vi "3_AdvancedDemo_MHT3.vi"() -> ()   [LabVIEW 2017]
uses:
  Types/MH_InputChannel.ctl
  Types/MH_UIThread_Cmds.ctl
  Types/MH_UIThread_Data.ctl
  _lib/PQ/MultiHarp/MH_InitInfo.ctl
  Types/MH_SetInpChanData.ctl
  Types/MH_SetInpChanCmds.ctl
  Types/MH_DataProcThread_QData.ctl
  Types/MH_DataProcThread_QCmds.ctl
  Types/MH_VisThread_QData.ctl
  Types/MH_VisThread_QCmds.ctl
  Types/MH_VisThread_Data.ctl
  _lib/PQ/MultiHarp/MH_RefSource.ctl
  _lib/PQ/MultiHarp/MH_MeasMode.ctl
  <vilib>/Utility/error.llb/DialogType.ctl
  <vilib>/Utility/error.llb/Error Cluster From Error Code.vi
  _lib/PQ/MultiHarp/MH_LibVersion_global.vi
  _lib/PQ/MultiHarp/mhlib_x86_x64_UIThread.llb/MH_DllPath_global.vi
  <vilib>/ErrorRing/Error Ring.xnode
panel:
  in  "Settings":bool=TRUE
  in  "Run continuously":bool caption="Conti."
  in  "Start":bool
  in  "Scale":bool
  out "CountRates":i32[](graph)
  in  "AllChannels":T1={"Enable"=TRUE, "Offset"=0, "Level"=-100, "Edge"=0, "DeadTime"=1000, "UseDeadTime"=FALSE, "SetEnableAllChan"=TRUE, "SetEdgeAllChan"=TRUE, "SetLevelAllChan"=TRUE, "SetOffsetAllChan"=TRUE, "SetUseDTAllChan"=TRUE, "SetDeadTAllChan"=TRUE} {"DeadTime" min=800 max=160000 step=1; "Edge" items=["falling", "rising"]; "Offset" min=-100000 max=100000 step=80; "Level" min=-1200 max=1200 step=1}
  in  "HistoAcqTime":dbl=1.0 caption="Hist.Int.Time  s" min=0.1 max=360000.0 step=0.1
  in  "AcqTime":i32=360000000 caption="T3Acqu.       ms" min=1 max=360000 step=1
  in  "Binning":i32(ring) caption="Resol.            ps" items=["80", "160", "320", "640", "1280", "2560", "5120", "10240", "20480", "40960", "81920", "163840", "327680", "655360", "1310720", "2621440", "5242880", "10485760", "20971520", "41943040", "83886080", "167772160", "335544320"]
  in  "HistoOffset":i32 caption="Offset            ns" min=0 max=100000000 step=1
  out "DeltaT":dbl=6.553665536655367 caption="T.Tr.Resol.   ms" format="%.2f"
  in  "BitShift":i32=15 min=0 max=32 step=1
  in  "OvlLevel":u32=4294967295 caption="Ovl.Level" min=1024 max=65536 step=1024
  in  "StopOvl.":bool=TRUE
  out "TTraceGraph":T2(graph)={49.38852226226715, "Resolution"=0.00655367864414373, "Histogram"=[]}
  out "HistoGraph":cluster{dbl, "Resol":dbl, "Histos":u32[][]}(graph)={0.0, "Resol"=0.08, "Histos"=[]}
  in  "SyncDeadTime":i32=1000 caption="Dead T.   ps" min=800 max=160000 step=1
  in  "UseDeadTime":bool caption="Use DT."
  in  "SyncEdge":i32(ring) caption="Edge" items=["falling", "rising"]
  in  "SyncDivider":i32(ring) caption="Divider" items=["1", "2", "4", "8", "16"]
  in  "SyncOffset":i32 caption="Offset      ps" min=-100000 max=100000 step=80
  in  "SyncLevel":i32=-100 caption="Level      mV" min=-1200 max=1200 step=1
  in  "Channels":T3[](array[typedef])=[{"Name"="Inp.Chan 1", "Enable"=TRUE, "Edge"=0, "Level"=-100, "Offset"=0, "UseDeadTime"=FALSE, "DeadTime"=1000}, {"Name"="Inp.Chan 2", "Enable"=TRUE, "Edge"=0, "Level"=-100, "Offset"=0, "UseDeadTime"=FALSE, "DeadTime"=1000}, {"Name"="Inp.Chan 3", "Enable"=TRUE, "Edge"=0, "Level"=-100, "Offset"=0, "UseDeadTime"=FALSE, "DeadTime"=1000}, {"Name"="Inp.Chan 4", "Enable"=TRUE, "Edge"=0, "Level"=-100, "Offset"=0, "UseDeadTime"=FALSE, "DeadTime"=1000}, {"Name"="Inp.Chan 5", "Enable"=TRUE, "Edge"=0, "Level"=-100, "Offset"=0, "UseDeadTime"=FALSE, "DeadTime"=1000}, {"Name"="Inp.Chan 6", "Enable"=TRUE, "Edge"=0, "Level"=-100, "Offset"=0, "UseDeadTime"=FALSE, "DeadTime"=1000}, {"Name"="Inp.Chan 7", "Enable"=TRUE, "Edge"=0, "Level"=-100, "Offset"=0, "UseDeadTime"=FALSE, "DeadTime"=1000}, {"Name"="Inp.Chan 8", "Enable"=TRUE, "Edge"=0, "Level"=-100, "Offset"=0, "UseDeadTime"=FALSE, "DeadTime"=1000}, {"Name"="Inp.Chan 9", "Enable"=TRUE, "Edge"=0, "Level"=-100, "Offset"=0, "UseDeadTime"=FALSE, "DeadTime"=1000}, {"Name"="Inp.Chan 10", "Enable"=TRUE, "Edge"=0, "Level"=-100, "Offset"=0, "UseDeadTime"=FALSE, "DeadTime"=1000}, {"Name"="Inp.Chan 11", "Enable"=TRUE, "Edge"=0, "Level"=-100, "Offset"=0, "UseDeadTime"=FALSE, "DeadTime"=1000}, {"Name"="Inp.Chan 12", "Enable"=TRUE, "Edge"=0, "Level"=-100, "Offset"=0, "UseDeadTime"=FALSE, "DeadTime"=1000}, {"Name"="Inp.Chan 13", "Enable"=TRUE, "Edge"=0, "Level"=-100, "Offset"=0, "UseDeadTime"=FALSE, "DeadTime"=1000}, {"Name"="Inp.Chan 14", "Enable"=TRUE, "Edge"=0, "Level"=-100, "Offset"=0, "UseDeadTime"=FALSE, "DeadTime"=1000}, {"Name"="Inp.Chan 15", "Enable"=TRUE, "Edge"=0, "Level"=-100, "Offset"=0, "UseDeadTime"=FALSE, "DeadTime"=1000}, {"Name"="Inp.Chan 16", "Enable"=TRUE, "Edge"=0, "Level"=-100, "Offset"=0, "UseDeadTime"=FALSE, "DeadTime"=1000}] {"DeadTime" min=800 max=160000 step=1; "Edge" items=["falling", "rising"]; "Offset" min=-100000 max=100000 step=80; "Level" min=-1200 max=1200 step=1}
  out "SyncRate":string="Sync Rate: 4999940 cps\n"
  out "OverRun":bool caption="Overrun:"
  out "Status":string="Elements in Q: 0"
  # "All Channels"
  # "Acquisition"
  # "Sync"
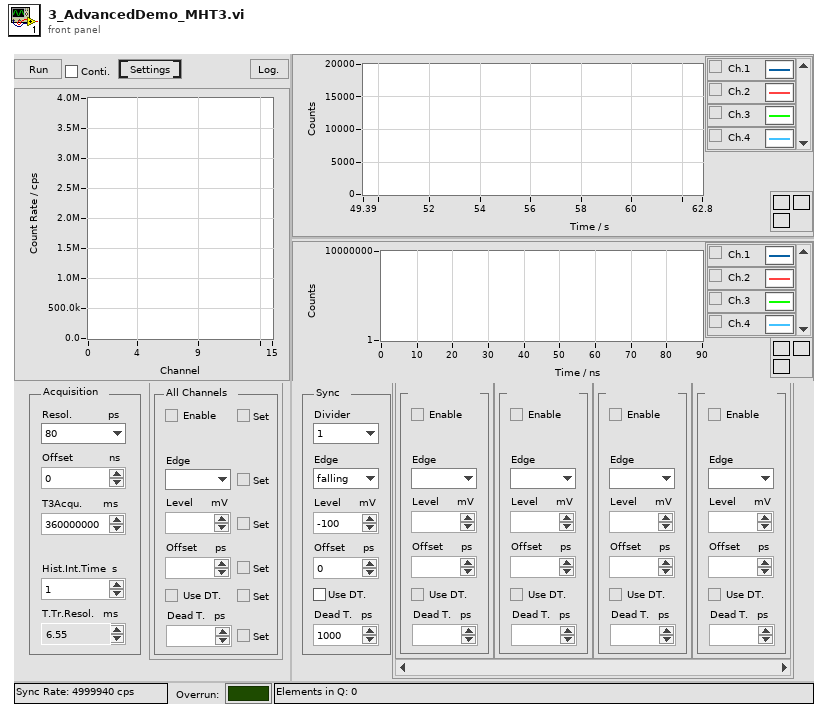
[diagram p1: front panel]
types:
  T1 = cluster{"Enable":bool, "Offset":i32, "Level":i32, "Edge":i32, "DeadTime":i32, "UseDeadTime":bool, "SetEnableAllChan":bool, "SetEdgeAllChan":bool, "SetLevelAllChan":bool, "SetOffsetAllChan":bool, "SetUseDTAllChan":bool, "SetDeadTAllChan":bool}
  T2 = cluster{dbl, "Resolution":dbl, "Histogram":u32[][]}
  T3 = typedef "MH_InputChannel.ctl" = cluster{"Name":string, "Enable":bool, "Edge":i32, "Level":i32, "Offset":i32, "UseDeadTime":bool, "DeadTime":i32}
  T4 = typedef "MH_DataProcThread_QCmds.ctl" = enum16{"Exit", "Proc", "Init", "SetShift", "SetNumChannels", "SetHistAcqTime"}
  T5 = typedef "MH_VisThread_Data.ctl" = cluster{"Resol":dbl, "DeltaT":dbl, "NumChannels":i32}
  T6 = typedef "MH_VisThread_QData.ctl" = cluster{"Histos":u32[][], "Cmd":T7, "TimeTrace":u32[][], "Bin":i32, "Total bin":u64, "Status":string, "Resol":dbl, "DeltaT":dbl, "nChannels":i32}
  T7 = typedef "MH_VisThread_QCmds.ctl" = enum16{"_none_", "Resol", "nChannels", "DeltaT", "Histo", "TTrace", "Status"}
  T8 = typedef "MH_DataProcThread_QData.ctl" = cluster{"Cmd":T4, "nActual":i32, "Buffer":u32[], "TickCount":u32, "Param":i32}
  T9 = typedef "MH_UIThread_Data.ctl" = cluster{"Init Info":T10, "DevIdx":i32, "SyncDivider":i32, "SyncOffset":i32, "SyncLevel":i32, "Channels":T3[], "CurrentChannels":i32[], "AcqTime":i32, "Binning":i32, "HistoOffset":i32, "HistoLen":i32, "StopOvl.":bool, "OvlLevel":u32, "SyncEdge":i32, "StartMeas":bool, "HistoLength":i32, "Resolution":dbl, "Run cont.":bool, "Status":string, "SyncRate":i32, "BitShift":i32, "HistoAcqTime":dbl, "SyncRateStart":i32, "UseDeadTime":bool, "SyncDeadTime":i32, "SetInpChan":T11[]}
  T10 = typedef "MH_InitInfo.ctl" = cluster{"Library Version":string, "Serial No.":string, "Model":string, "Partnum":string, "Version":string, "features":i32, "nchannels":i32, "Base Resolution":dbl, "Bin Steps":i32}
  T11 = typedef "MH_SetInpChanData.ctl" = cluster{"Channel":i32, "Cmds":T12[], "Changed":cluster{"Name":bool, "Enable":bool, "Edge":bool, "Level":bool, "Offset":bool, "UseDeadTime":bool, "DeadTime":bool}}
  T12 = typedef "MH_SetInpChanCmds.ctl" = enum16{"SetInpChanEnable", "SetInpChanOffset", "SetInpChanDeadTime", "SetInpChanTrg"}
  T13 = typedef "MH_UIThread_Cmds.ctl" = enum16{"Idle", "Init", "SetInpChan", "SetSyncDivider", "SetSyncTrg", "SetSyncOffset", "SetSyncDeadTime", "SetBinning", "SetHistoOffset", "SetHistoLen", "SetStopOvl", "SetBitShift", "SetHistoAcqTime", "GetRates", "GetAllRates", "StartMeas", "StopMeas", "AbortMeas", "GetResolution", "GetHistos", "GetAllHistos", "ReadFiFo", "WriteStatus", "Resize", "EnableControls", "DisableControls", "Error", "Exit"}
  T14 = enum8{"Enabled", "Disabled", "Disabled and Grayed Out"}
  T15 = cluster{"[0]":bool, "[1]":bool, "[2]":bool, "[3]":bool, "[4]":bool, "[5]":bool}
  T16 = typedef "MH_MeasMode.ctl" = i32
  T17 = typedef "MH_RefSource.ctl" = enum16{"INTERNAL", "EXTERNAL_10MHZ", "WR_MASTER_GENERIC", "WR_SLAVE_GENERIC", "WR_GRANDM_GENERIC", "EXTN_GPS_PPS", "EXTN_GPS_PPS_UART", "WR_MASTER_MHARP", "WR_SLAVE_MHARP", "WR_GRANDM_MHARP"}
  T18 = typedef "DialogType.ctl" = u16
  T19 = cluster{"T0":dbl, "dt":dbl, "TimeTrace_out":u32[][]}
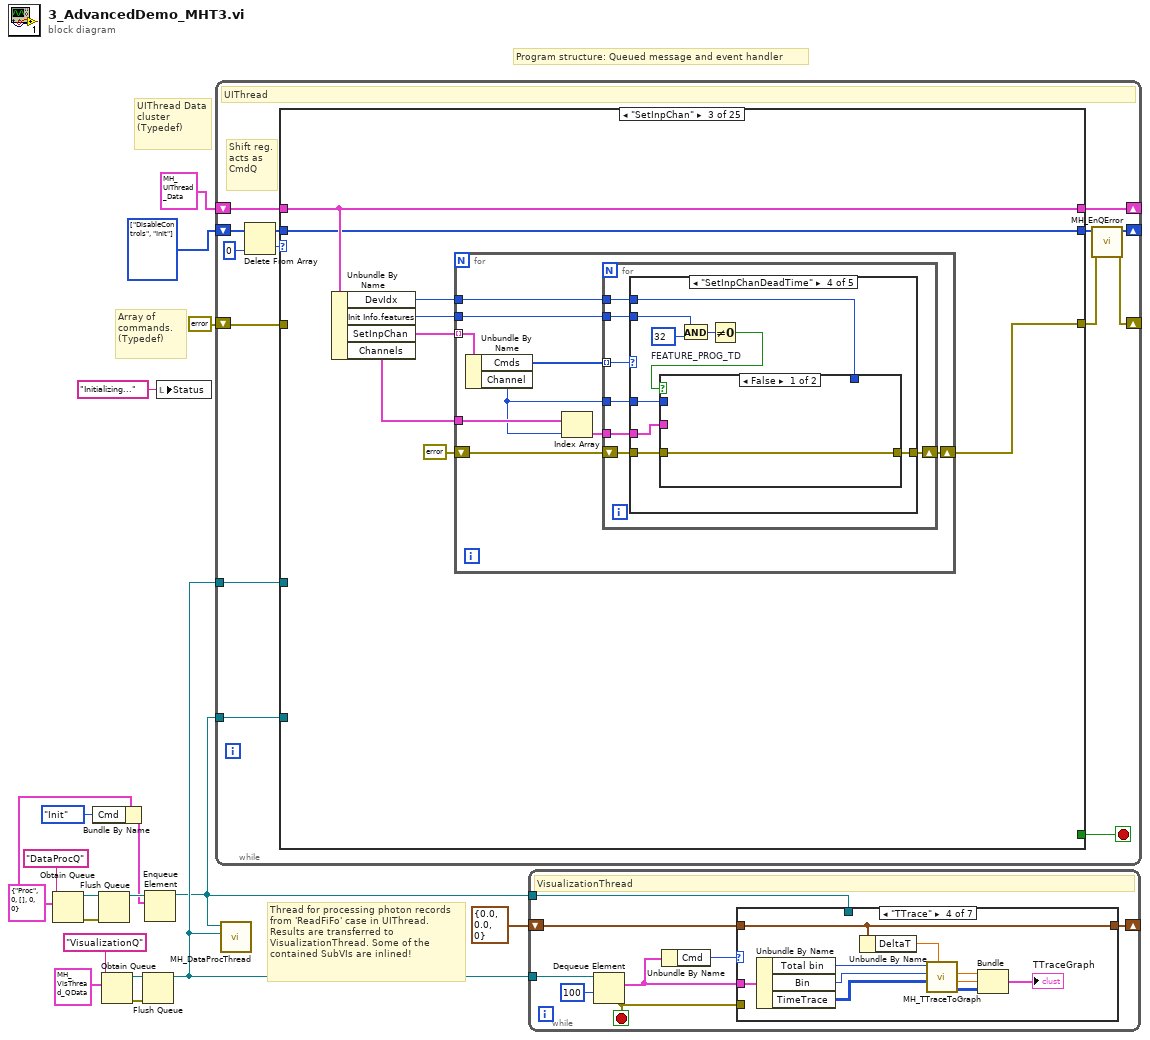
[diagram p0: block diagram]
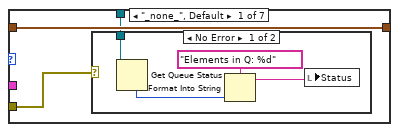
[diagram p2: hidden frame]
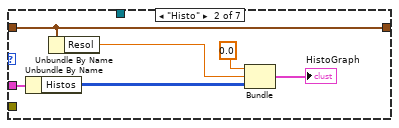
[diagram p4: hidden frame]
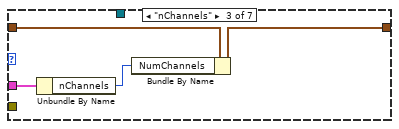
[diagram p5: hidden frame]
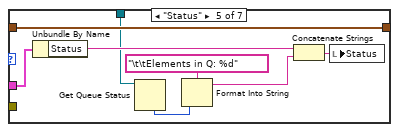
[diagram p6: hidden frame]
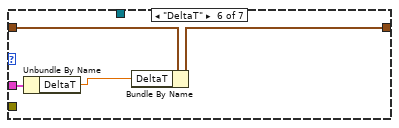
[diagram p7: hidden frame]
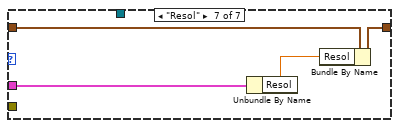
[diagram p8: hidden frame]
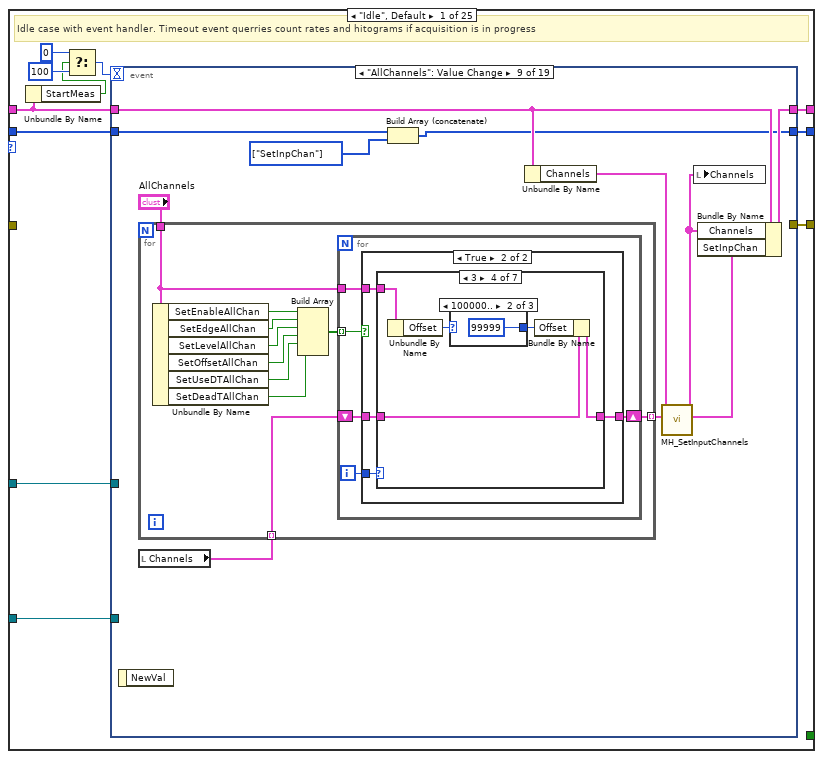
[diagram p9: hidden frame]
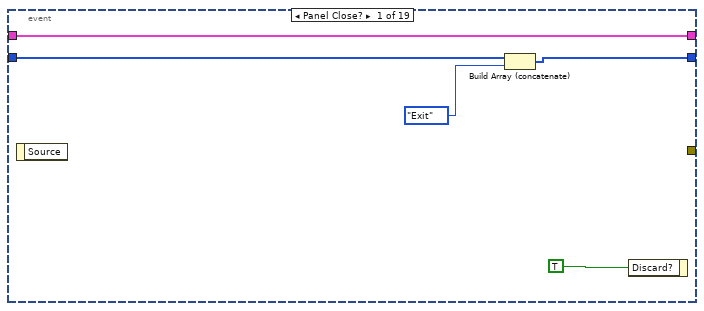
[diagram p10: hidden frame]
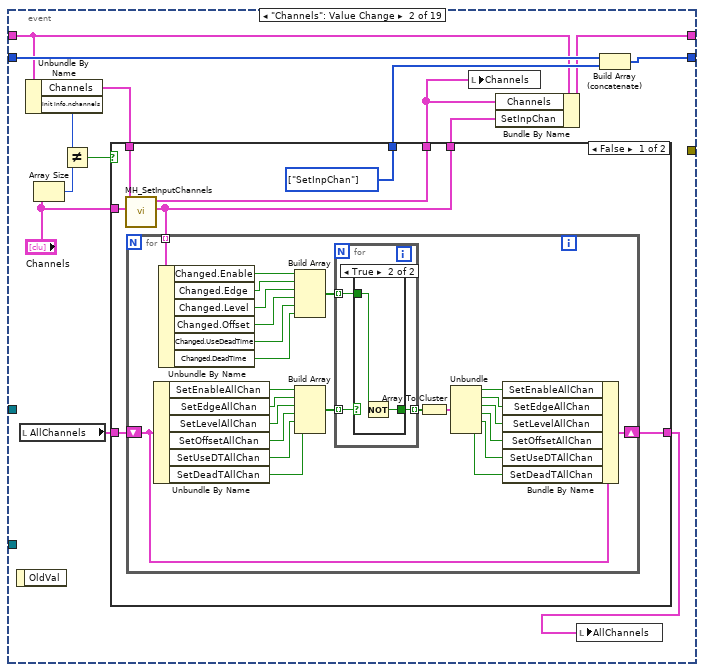
[diagram p11: hidden frame]
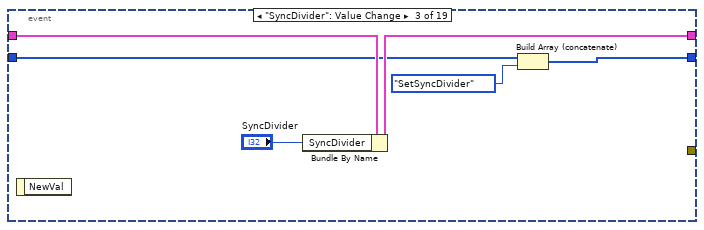
[diagram p14: hidden frame]
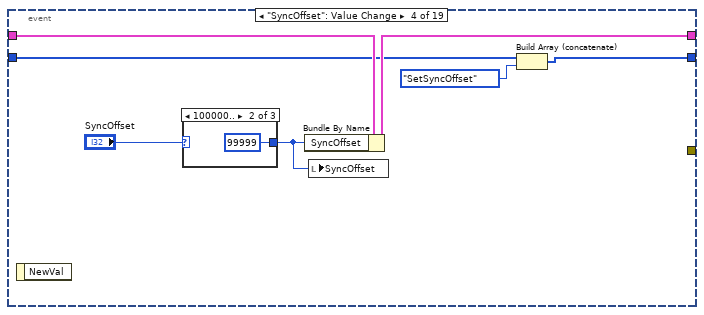
[diagram p15: hidden frame]
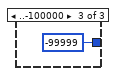
[diagram p17: hidden frame]
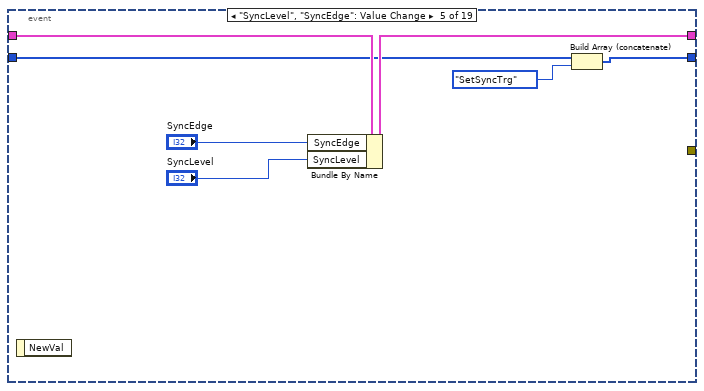
[diagram p18: hidden frame]
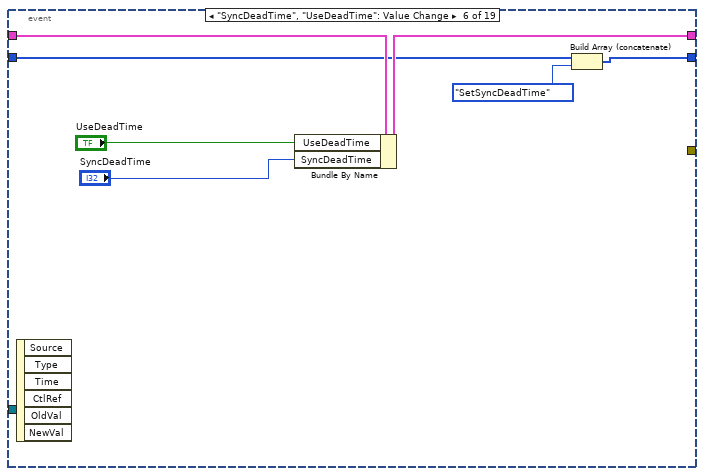
[diagram p19: hidden frame]
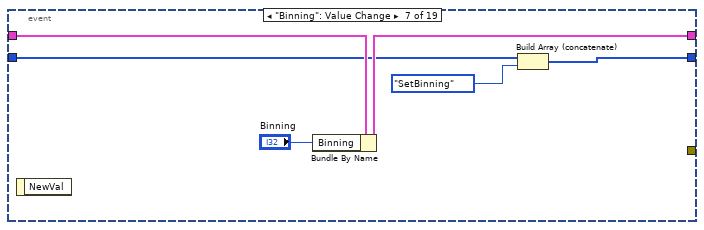
[diagram p20: hidden frame]
diagram:
  w4 = T8 {"Cmd"=enum."Proc", "nActual"=0, "Buffer"=[], "TickCount"=0, "Param"=0} ("MH_DataProcThread_QData")
  w17 = T13[] [enum."DisableControls", enum."Init"] items=["Idle", "Init", "SetInpChan", "SetSyncDivider", "SetSyncTrg", "SetSyncOffset", "SetSyncDeadTime", "SetBinning", "SetHistoOffset", "SetHistoLen", "SetStopOvl", "SetBitShift", "SetHistoAcqTime", "GetRates", "GetAllRates", "StartMeas", "StopMeas", "AbortMeas", "GetResolution", "GetHistos", "GetAllHistos", "ReadFiFo", "WriteStatus", "Resize", "EnableControls", "DisableControls", "Error", "Exit"]
  # "Thread for processing photon records from 'ReadFiFo' case in UIThread. Results are transferred to VisualizationThread. Some of the contained SubVIs are inlined!"
  # "Array of commands.\n(Typedef)"
  # "Program structure: Queued message and event handler"
  # "UIThread Data cluster\n(Typedef)"
  n1 = Obtain Queue(name (unnamed)="DataProcQ", element data type=w4) -> (queue out=w14:refnum<queue>, error out=w13:errorcluster)  [unwired: 3 in, 1 out]
  n2 = Bundle By Name(cluster=w4, "Cmd"=MH_DataProcThread_QCmds."Init") -> (w2:T8)
  n3 = Flush Queue(queue=w14, error in (no error)=w13) -> (queue out=w5:refnum<queue>)  [unwired: 2 out]
  n4 = Obtain Queue(name (unnamed)="VisualizationQ", element data type=T6 {"Histos"=[], "Cmd"=enum."_none_", "TimeTrace"=[], "Bin"=0, "Total bin"=0, "Status"="", "Resol"=0.0, "DeltaT"=0.0, "nChannels"=0} ("MH_GUIThread_QData")) -> (queue out=w12:refnum<queue>, error out=w11:errorcluster)  [unwired: 3 in, 1 out]
  n5 = Flush Queue(queue=w12, error in (no error)=w11) -> (queue out=w7:refnum<queue>)  [unwired: 2 out]
  n6 = Enqueue Element(queue=w5, element=w2) -> (queue out=w1:refnum<queue>)  [unwired: 2 in, 2 out]
  n7 = local write "Status"("Initializing..." ("Status")) -> ()
  n8 = while {
    shift-right: [w21] -> _
    shift-left: w17 -> [w28]
    shift-right: [w31] -> _
    shift-left: T9 {"Init Info"={"Library Version"="", "Serial No."="", "Model"="", "Partnum"="", "Version"="", "features"=0, "nchannels"=0, "Base Resolution"=0.0, "Bin Steps"=0}, "DevIdx"=0, "SyncDivider"=1, "SyncOffset"=0, "SyncLevel"=50, "Channels"=[], "CurrentChannels"=[], "AcqTime"=1, "Binning"=1, "HistoOffset"=1, "HistoLen"=1024, "StopOvl."=FALSE, "OvlLevel"=1024, "SyncEdge"=10, "StartMeas"=FALSE, "HistoLength"=0, "Resolution"=0.0, "Run cont."=FALSE, "Status"="", "SyncRate"=0, "BitShift"=0, "HistoAcqTime"=0.0, "SyncRateStart"=0, "UseDeadTime"=FALSE, "SyncDeadTime"=800, "SetInpChan"=[]} -> [w30]
    shift-right: [w23] -> _
    shift-left: errorcluster {"status"=FALSE, "code"=0, "source"=""} ("error IO") -> [w29]
    tunnel: w1 -> [w20]
    tunnel: w7 -> [w19]
    stop <- w32 stop-if-true
    # "Shift reg.\nacts as\nCmdQ"
    # "UIThread"
    n9 = Delete From Array(array=w28, index=0) -> (deleted portion=w26:T13, array with subset deleted=w25:T13[])  [unwired: 1 in]
    n10 = case shown="\"SetInpChan\"" w26 {
      tunnel: [w43 w353 w376 w438 w447 w459 w465 w472 w480 w487 w507 w519 w522 w594 w617 w622 w635 w652 w653 w679 w692 w699 w711 w717 w723] -> w22
      tunnel: [_ _ _ _ _ _ _ _ _ _ _ _ _ _ _ _ _ _ _ _ _ _ _ _ TRUE] -> w32
      tunnel: [w42 w334 w377 w440 w448 w460 w469 w476 w481 w488 w492 w509 w531 w586 w609 w625 w637 w648 w663 w678 w680 w698 w710 w718 w726] -> w31
      tunnel: w30 -> [w39 w339 w377 w440 w448 w460 w469 w476 w481 w488 w492 w509 w521 w587 w610 w626 w638 w649 w663 w678 w680 w698 w710 w718 w726]
      tunnel: [w40 w356 w371 w436 w446 w458 w468 w475 w479 w486 _ _ w527 w593 w620 w628 w640 w650 w658 _ _ _ _ _ w724] -> w24
      tunnel: w29 -> [_ _ _ _ _ _ _ _ _ _ _ _ _ _ _ _ _ _ _ _ _ _ _ w719 _]
      tunnel: w25 -> [w41 w355 w376 w438 w447 w459 w465 w471 w480 w487 w507 w519 w523 w594 w618 w623 w635 w652 w654 w679 w692 w699 w711 _ w723]
      tunnel: w20 -> [w34 w332 _ _ _ _ _ _ _ _ w493 w510 _ _ w614 _ _ _ w655 _ _ _ _ _ w722]
      tunnel: w19 -> [w33 w325 _ _ _ _ _ _ _ _ w494 _ _ _ _ _ _ w645 _ _ _ _ _ _ w721]
      frame "Idle", Default {
        # "Idle case with event handler. Timeout event querries count rates and hitograms if acquisition is in progress"
        n11 = Unbundle By Name(w39) -> ("StartMeas"=w37:bool)
        n12 = Select(t=0, s=w37, f=100) -> (s? t:f=w36:i32)
        n13 = event shown="[8] \"AllChannels\": Value Change" {
          selector: _ -> [_ _ _ _ _ _ _ _ _ _ _ _ _ _ _ _ _ _ _]
          dyn-events: _ -> [_ _ _ _ _ _ _ _ _ _ _ _ _ _ _ _ _ _ _]
          timeout: w36 -> [_ _ _ _ _ _ _ _ _ _ _ _ _ _ _ _ _ _ _]
          tunnel: [w44 w61 w103 w111 w120 w128 w134 w140 w145 w205 w210 w217 w232 w250 w262 w280 w286 w294 w304] -> w43
          tunnel: [w47 w53 w107 w114 w124 w131 w137 w143 w150 w207 w213 w220 w231 w254 w261 w278 w285 w293 w307] -> w42
          tunnel: w39 -> [w47 w54 w108 w115 w125 w132 w138 w144 w151 w208 w214 w221 w231 w255 w259 w279 w285 w293 w307]
          tunnel: w41 -> [w46 w62 w105 w113 w122 w130 w136 w142 w146 w205 w211 w219 w233 w251 w263 w280 w286 w294 w305]
          tunnel: [_ _ _ _ _ _ _ _ _ _ _ _ w227 _ _ _ _ _ _] -> w40
          tunnel: w34 -> [_ _ _ _ _ _ _ _ _ _ _ _ _ _ _ _ _ _ _]
          tunnel: w33 -> [_ _ _ _ _ _ _ _ _ _ _ _ _ _ _ _ _ _ _]
          event Panel Close? {
            n14 = event-data() -> ()  [unwired: 1 in, 1 out]
            n15 = Build Array (concatenate)(w46, MH_UIThread_Cmds."Exit") -> (w44:T13[])
            n16 = event-data("Discard?"=TRUE) -> ()  [unwired: 1 in, 1 out]
          }
          event "Channels": Value Change {
            n17 = event-data() -> ()  [unwired: 1 in, 1 out]
            n18 = local read "AllChannels"() -> (w49:T1)
            n19 = Unbundle By Name(w54) -> ("Channels"=w56:T3[], "Init Info.nchannels"=w58:i32)
            n20 = Array Size(array="Channels") -> (size(s)=w59:i32)
            n21 = Not Equal?(x=w58, y=w59) -> (x != y?=w57:bool)
            n22 = case shown="False" w57 {
              tunnel: "Channels" -> [w68 _]
              tunnel: [w67 w102] -> w51
              tunnel: w56 -> [w69 w102]
              tunnel: [w65 _] -> w52
              tunnel: [w66 _] -> w55
              tunnel: w49 -> [w64 w101]
              tunnel: [w63 w101] -> w50
              frame False {
                w66 = T13[] [enum."SetInpChan"] items=["Idle", "Init", "SetInpChan", "SetSyncDivider", "SetSyncTrg", "SetSyncOffset", "SetSyncDeadTime", "SetBinning", "SetHistoOffset", "SetHistoLen", "SetStopOvl", "SetBitShift", "SetHistoAcqTime", "GetRates", "GetAllRates", "StartMeas", "StopMeas", "AbortMeas", "GetResolution", "GetHistos", "GetAllHistos", "ReadFiFo", "WriteStatus", "Resize", "EnableControls", "DisableControls", "Error", "Exit"] ("array")
                n23 = call "MH_SetInputChannels.vi"("Channels new"=w68, "Channels old"=w69) -> ("SetInpChan"=w65:T11[], "Channels"=w67:T3[])  [unwired: 8 in]
                n24 = for {
                  tunnel: w65 -> [w94] mode=indexing
                  shift-right: [w76] -> w63
                  shift-left: w64 -> [w78]
                  n25 = Unbundle By Name(w78) -> ("SetEnableAllChan"=w87:bool, "SetEdgeAllChan"=w86:bool, "SetLevelAllChan"=w85:bool, "SetOffsetAllChan"=w84:bool, "SetUseDTAllChan"=w83:bool, "SetDeadTAllChan"=w82:bool)
                  n26 = Unbundle By Name(w94) -> ("Changed.Enable"=w93:bool, "Changed.Edge"=w92:bool, "Changed.Level"=w91:bool, "Changed.Offset"=w90:bool, "Changed.UseDeadTime"=w89:bool, "Changed.DeadTime"=w88:bool)
                  n27 = Build Array(w93, w92, w91, w90, w89, w88) -> (w80:bool[])
                  n28 = Build Array(w87, w86, w85, w84, w83, w82) -> (w81:bool[])
                  n29 = for {
                    tunnel: w81 -> [w97] mode=indexing
                    tunnel: w80 -> [w95] mode=indexing
                    tunnel: [w96] -> w79 mode=indexing
                    n30 = case shown="True" w97 {
                      selector: w97 -> [w98 _]
                      tunnel: [w98 w99] -> w96
                      tunnel: w95 -> [_ w100]
                      frame False {
                      }
                      frame True {
                        n31 = Not(x=w100) -> (.not. x?=w99:bool)
                      }
                    }
                  }
                  n32 = Array To Cluster(array=w79) -> (cluster=w77:T15)
                  n33 = Unbundle(w77) -> ("[0]"=w75:bool, "[1]"=w74:bool, "[2]"=w73:bool, "[3]"=w72:bool, "[4]"=w71:bool, "[5]"=w70:bool)
                  n34 = Bundle By Name(cluster=w78, "SetEnableAllChan"=w75, "SetEdgeAllChan"=w74, "SetLevelAllChan"=w73, "SetOffsetAllChan"=w72, "SetUseDTAllChan"=w71, "SetDeadTAllChan"=w70) -> (w76:T1)
                }
              }
              frame True {
              }
            }
            n35 = local write "Channels"(w51) -> ()
            n36 = Bundle By Name(cluster=w54, "Channels"=w51, "SetInpChan"=w52) -> (w53:T9)
            n37 = local write "AllChannels"(w50) -> ()
            n38 = Build Array (concatenate)(w62, w55) -> (w61:T13[])
          }
          event "SyncDivider": Value Change {
            n39 = event-data() -> ()  [unwired: 1 in, 1 out]
            n40 = Bundle By Name(cluster=w108, "SyncDivider"="SyncDivider") -> (w107:T9)
            n41 = Build Array (concatenate)(w105, MH_UIThread_Cmds."SetSyncDivider") -> (w103:T13[])
          }
          event "SyncOffset": Value Change {
            n42 = event-data() -> ()  [unwired: 1 in, 1 out]
            n43 = case shown="100000.." "SyncOffset" {
              selector: "SyncOffset" -> [w116 _ _]
              tunnel: [w116 99999 ("SyncOffset") -99999 ("SyncOffset")] -> w109
              frame Default {
              }
              frame 100000.. {
              }
              frame ..-100000 {
              }
            }
            n44 = Bundle By Name(cluster=w115, "SyncOffset"=w109) -> (w114:T9)
            n45 = local write "SyncOffset"(w109) -> ()
            n46 = Build Array (concatenate)(w113, MH_UIThread_Cmds."SetSyncOffset") -> (w111:T13[])
          }
          event "SyncLevel", "SyncEdge": Value Change {
            n47 = event-data() -> ()  [unwired: 1 in, 1 out]
            n48 = Bundle By Name(cluster=w125, "SyncEdge"="SyncEdge", "SyncLevel"="SyncLevel") -> (w124:T9)
            n49 = Build Array (concatenate)(w122, MH_UIThread_Cmds."SetSyncTrg") -> (w120:T13[])
          }
          event "SyncDeadTime", "UseDeadTime": Value Change {
            n50 = event-data() -> ()  [unwired: 1 in, 6 out]
            n51 = Bundle By Name(cluster=w132, "UseDeadTime"="UseDeadTime", "SyncDeadTime"="SyncDeadTime") -> (w131:T9)
            n52 = Build Array (concatenate)(w130, MH_UIThread_Cmds."SetSyncDeadTime") -> (w128:T13[])
          }
          event "Binning": Value Change {
            n53 = event-data() -> ()  [unwired: 1 in, 1 out]
            n54 = Bundle By Name(cluster=w138, "Binning"="Binning") -> (w137:T9)
            n55 = Build Array (concatenate)(w136, MH_UIThread_Cmds."SetBinning") -> (w134:T13[])
          }
          event "HistoOffset": Value Change {
            n56 = event-data() -> ()  [unwired: 1 in, 1 out]
            n57 = Bundle By Name(cluster=w144, "HistoOffset"="HistoOffset") -> (w143:T9)
            n58 = Build Array (concatenate)(w142, MH_UIThread_Cmds."SetHistoOffset") -> (w140:T13[])
          }
          event "AllChannels": Value Change {
            w147 = T13[] [enum."SetInpChan"] items=["Idle", "Init", "SetInpChan", "SetSyncDivider", "SetSyncTrg", "SetSyncOffset", "SetSyncDeadTime", "SetBinning", "SetHistoOffset", "SetHistoLen", "SetStopOvl", "SetBitShift", "SetHistoAcqTime", "GetRates", "GetAllRates", "StartMeas", "StopMeas", "AbortMeas", "GetResolution", "GetHistos", "GetAllHistos", "ReadFiFo", "WriteStatus", "Resize", "EnableControls", "DisableControls", "Error", "Exit"] ("array")
            n59 = event-data() -> ()  [unwired: 1 in, 1 out]
            n60 = local read "Channels"() -> (w154:T3[])
            n61 = for {
              tunnel: w154 -> [w158] mode=indexing
              tunnel: "AllChannels" -> [w157]
              tunnel: [w156] -> w153 mode=indexing
              n62 = Unbundle By Name(w157) -> ("SetEnableAllChan"=w159:bool, "SetEdgeAllChan"=w160:bool, "SetLevelAllChan"=w161:bool, "SetOffsetAllChan"=w162:bool, "SetUseDTAllChan"=w163:bool, "SetDeadTAllChan"=w164:bool)
              n63 = Build Array(w159, w160, w161, w162, w163, w164) -> (w165:bool[])
              n64 = for {
                tunnel: w165 -> [w170] mode=indexing
                shift-right: [w167] -> w156
                shift-left: w158 -> [w168]
                tunnel: w157 -> [w166]
                i -> [w169]
                n65 = case shown="True" w170 {
                  tunnel: w169 -> [_ w175]
                  tunnel: w166 -> [_ w174]
                  tunnel: w168 -> [w171 w173]
                  tunnel: [w171 w172] -> w167
                  frame False {
                  }
                  frame True {
                    n66 = case shown="3" w175 {
                      tunnel: w174 -> [w179 w183 w187 w192 w199 w203 _]
                      tunnel: w173 -> [w178 w182 w186 w191 w198 w202 w204]
                      tunnel: [w176 w180 w184 w190 w196 w200 w204] -> w172
                      frame 0 {
                        n67 = Unbundle By Name(w179) -> ("Enable"=w177:bool)
                        n68 = Bundle By Name(cluster=w178, "Enable"=w177) -> (w176:T3)
                      }
                      frame 1 {
                        n69 = Unbundle By Name(w183) -> ("Edge"=w181:i32)
                        n70 = Bundle By Name(cluster=w182, "Edge"=w181) -> (w180:T3)
                      }
                      frame 2 {
                        n71 = Unbundle By Name(w187) -> ("Level"=w185:i32)
                        n72 = Bundle By Name(cluster=w186, "Level"=w185) -> (w184:T3)
                      }
                      frame 3 {
                        n73 = Unbundle By Name(w192) -> ("Offset"=w189:i32)
                        n74 = case shown="100000.." w189 {
                          selector: w189 -> [w193 _ _]
                          tunnel: [w193 99999 ("SyncOffset") -99999 ("SyncOffset")] -> w188
                          frame Default {
                          }
                          frame 100000.. {
                          }
                          frame ..-100000 {
                          }
                        }
                        n75 = Bundle By Name(cluster=w191, "Offset"=w188) -> (w190:T3)
                      }
                      frame 4 {
                        n76 = Unbundle By Name(w199) -> ("UseDeadTime"=w197:bool)
                        n77 = Bundle By Name(cluster=w198, "UseDeadTime"=w197) -> (w196:T3)
                      }
                      frame 5 {
                        n78 = Unbundle By Name(w203) -> ("DeadTime"=w201:i32)
                        n79 = Bundle By Name(cluster=w202, "DeadTime"=w201) -> (w200:T3)
                      }
                      frame Default {
                      }
                    }
                  }
                }
              }
            }
            n80 = Build Array (concatenate)(w146, w147) -> (w145:T13[])
            n81 = Unbundle By Name(w151) -> ("Channels"=w152:T3[])
            n82 = call "MH_SetInputChannels.vi"("Channels new"=w153, "Channels old"=w152) -> ("SetInpChan"=w148:T11[], "Channels"=w149:T3[])  [unwired: 8 in]
            n83 = local write "Channels"(w149) -> ()
            n84 = Bundle By Name(cluster=w151, "Channels"=w149, "SetInpChan"=w148) -> (w150:T9)
          }
          event "AcqTime": Value Change {
            n85 = event-data() -> ()  [unwired: 1 in, 1 out]
            n86 = Bundle By Name(cluster=w208, "AcqTime"="AcqTime") -> (w207:T9)
          }
          event "HistoAcqTime": Value Change {
            n87 = event-data() -> ()  [unwired: 1 in, 1 out]
            n88 = Bundle By Name(cluster=w214, "HistoAcqTime"="HistoAcqTime") -> (w213:T9)
            n89 = Build Array (concatenate)(w211, MH_UIThread_Cmds."SetHistoAcqTime") -> (w210:T13[])
          }
          event "OvlLevel", "StopOvl.": Value Change {
            n90 = event-data() -> ()  [unwired: 1 in, 1 out]
            n91 = Bundle By Name(cluster=w221, "StopOvl."="StopOvl.", "OvlLevel"="OvlLevel") -> (w220:T9)
            n92 = Build Array (concatenate)(w219, MH_UIThread_Cmds."SetStopOvl") -> (w217:T13[])
          }
          event Timeout {
            n93 = event-data() -> ()  [unwired: 1 in, 1 out]
            n94 = Unbundle By Name(w231) -> ("DevIdx"=w229:i32, "StartMeas"=w230:bool, "BitShift"=w226:i32, "SyncRate"=w225:i32)
            n95 = case shown="True" w230 {
              tunnel: w229 -> [_ w249]
              tunnel: [_ w247] -> w228
              tunnel: [_ w244] -> w227
              frame False {
              }
              frame True {
                w245 = T13[] [enum."ReadFiFo"] items=["Idle", "Init", "SetInpChan", "SetSyncDivider", "SetSyncTrg", "SetSyncOffset", "SetSyncDeadTime", "SetBinning", "SetHistoOffset", "SetHistoLen", "SetStopOvl", "SetBitShift", "SetHistoAcqTime", "GetRates", "GetAllRates", "StartMeas", "StopMeas", "AbortMeas", "GetResolution", "GetHistos", "GetAllHistos", "ReadFiFo", "WriteStatus", "Resize", "EnableControls", "DisableControls", "Error", "Exit"]
                w246 = T13[] [enum."StopMeas"] items=["Idle", "Init", "SetInpChan", "SetSyncDivider", "SetSyncTrg", "SetSyncOffset", "SetSyncDeadTime", "SetBinning", "SetHistoOffset", "SetHistoLen", "SetStopOvl", "SetBitShift", "SetHistoAcqTime", "GetRates", "GetAllRates", "StartMeas", "StopMeas", "AbortMeas", "GetResolution", "GetHistos", "GetAllHistos", "ReadFiFo", "WriteStatus", "Resize", "EnableControls", "DisableControls", "Error", "Exit"]
                n96 = call "MH_CTCStatus.vi"("devidx"=w249) -> ("error out"=w244:errorcluster, "ctcstatus"=w248:i32)  [unwired: 8 in, 1 out]
                n97 = Not Equal To 0?(x=w248) -> (x != 0?=w243:bool)
                n98 = Select(t=w246, s=w243, f=w245) -> (s? t:f=w247:T13[])
              }
            }
            n99 = call "CalcRate.vi"("Refresh(ms)"=u32 100) -> ("updated?"=w223:bool)  [unwired: 8 in, 2 out]
            n100 = case shown="True" w223 {
              tunnel: w226 -> [_ w236]
              tunnel: w225 -> [_ w235]
              tunnel: [_ MH_UIThread_Cmds."GetAllRates"] -> w224
              frame False {
              }
              frame True {
                n101 = To Double Precision Float(number=w235) -> (double precision float=w240:dbl)
                n102 = To Double Precision Float(number=w236) -> (double precision float=w241:dbl)
                n103 = Power Of 2(x=w241) -> (2^x=w239:dbl)
                n104 = Multiply(x=w239, y=1000.0) -> (x*y=w238:dbl)
                n105 = Divide(x=w238, y=w240) -> (x/y=w242:dbl)
                n106 = local write "DeltaT"(w242) -> ()
              }
            }
            n107 = Build Array (concatenate)(w233, w228, w224) -> (w232:T13[])
          }
          event "BitShift": Value Change {
            n108 = event-data() -> ()  [unwired: 1 in, 1 out]
            n109 = Bundle By Name(cluster=w255, "BitShift"="BitShift") -> (w254:T9)
            n110 = Build Array (concatenate)(w251, MH_UIThread_Cmds."SetBitShift") -> (w250:T13[])
          }
          event "Start": Value Change {
            n111 = event-data() -> ()  [unwired: 1 in, 1 out]
            n112 = Unbundle By Name(w259) -> ("SyncRate"=w258:i32)
            n113 = Greater Or Equal?(x=w258, y=10) -> (x >= y?=w256:bool)
            n114 = case shown="True" w256 {
              selector: w256 -> [w265 _]
              tunnel: w263 -> [w267 w276]
              tunnel: [w267 w274] -> w262
              tunnel: [w266 w273] -> w261
              tunnel: "Start" -> [_ w272]
              tunnel: w259 -> [w266 w268]
              frame False {
                n115 = local write "Start"(w265) -> ()
                n116 = One Button Dialog(message="SyncRate too low!!!" ("Status")) -> ()  [unwired: 1 in, 1 out]
              }
              frame True {
                w271 = T13[] [enum."SetBitShift", enum."SetHistoAcqTime", enum."StartMeas"] items=["Idle", "Init", "SetInpChan", "SetSyncDivider", "SetSyncTrg", "SetSyncOffset", "SetSyncDeadTime", "SetBinning", "SetHistoOffset", "SetHistoLen", "SetStopOvl", "SetBitShift", "SetHistoAcqTime", "GetRates", "GetAllRates", "StartMeas", "StopMeas", "AbortMeas", "GetResolution", "GetHistos", "GetAllHistos", "ReadFiFo", "WriteStatus", "Resize", "EnableControls", "DisableControls", "Error", "Exit"]
                n117 = Bundle By Name(cluster=w268, "StartMeas"=w272) -> (w273:T9)
                n118 = Build Array(MH_UIThread_Cmds."AbortMeas") -> (w269:T13[])
                n119 = Select(t=w271, s=w272, f=w269) -> (s? t:f=w275:T13[])
                n120 = Build Array (concatenate)(w276, w275) -> (w274:T13[])
              }
            }
          }
          event "Run continuously": Value Change {
            n121 = event-data() -> ()  [unwired: 1 in, 1 out]
            n122 = Bundle By Name(cluster=w279, "Run cont."="Run continuously") -> (w278:T9)
          }
          event "Scale": Value Change {
            n123 = event-data() -> ()  [unwired: 1 in, 1 out]
            n124 = Select(t=u8 0 ("Y Scale.Mapping Mode"), s="Scale", f=u8 1 ("Y Scale.Mapping Mode")) -> (s? t:f=w281:u8)
            n125 = property on="HistoGraph" class="WFGraph (strict)"("YScale.Mapping Mode"=w281) -> ()  [unwired: 2 in, 2 out]
          }
          event "Settings": Value Change {
            n126 = event-data() -> ()  [unwired: 1 in, 1 out]
            n127 = property on="Splitter" class="Splitter"() -> ("Position"=w292:i32)  [unwired: 2 in, 2 out]
            n128 = Select(t=300 ("PosT"), s="Settings", f=0 ("PosF")) -> (s? t:f=w289:i32)
            n129 = Subtract(x=w292, y=w289) -> (x-y=w288:i32)
            n130 = while {
              shift-right: [w303] -> _
              shift-left: w288 -> [w296]
              i -> [w302]
              stop <- w299 stop-if-true
              n131 = property on="Splitter 4" class="Splitter"("Position"=w296) -> (error out=w295:errorcluster)  [unwired: 2 in, 1 out]
              n132 = Greater Or Equal?(x=w302, y=10) -> (x >= y?=w300:bool)
              n133 = Decrement(x=w296) -> (x-1=w303:i32)
              n134 = Unbundle(w295) -> ("status"=w298:bool)  [unwired: 2 out]
              n135 = Not(x=w298) -> (.not. x?=w297:bool)
              n136 = Or(x=w297, y=w300) -> (x .or. y?=w299:bool)
            }
          }
          event Panel Resize {
            n137 = event-data() -> ()  [unwired: 1 in, 1 out]
            n138 = Build Array (concatenate)(w305, MH_UIThread_Cmds."Resize") -> (w304:T13[])
          }
        }
      }
      frame "Init" {
        w312 = 1000 ("SyncDeadTime")
        w313 = FALSE ("UseDeadTime")
        w315 = T16 3 items=["HIST"=0, "T2"=2, "T3"=3]  # Mode
        w317 = MH_RefSource."INTERNAL"  # refsource
        w323 = 1.0 ("HistoAcqTime")
        w324 = 15 ("Value (Signaling)")
        w341 = FALSE ("Run cont.")
        w343 = FALSE ("StartMeas")
        w344 = u32 4294967295 ("OvlLevel")
        w345 = TRUE ("StopOvl.")
        w346 = 360000000 ("AcqTime")
        w347 = 0 ("HistoOffset")
        w348 = 0 ("Binning")
        w349 = -100 ("SyncLevel")
        w350 = 0 ("SyncZeroX")
        w351 = 0 ("SyncOffset")
        w352 = 0 ("SyncDivider")
        w354 = T13[] [enum."SetSyncDivider", enum."SetSyncOffset", enum."SetSyncDeadTime", enum."SetSyncTrg", enum."SetInpChan", enum."SetBinning", enum."SetHistoOffset", enum."Resize", enum."EnableControls", enum."GetRates", enum."SetBitShift", enum."SetHistoAcqTime", enum."WriteStatus"] items=["Idle", "Init", "SetInpChan", "SetSyncDivider", "SetSyncTrg", "SetSyncOffset", "SetSyncDeadTime", "SetBinning", "SetHistoOffset", "SetHistoLen", "SetStopOvl", "SetBitShift", "SetHistoAcqTime", "GetRates", "GetAllRates", "StartMeas", "StopMeas", "AbortMeas", "GetResolution", "GetHistos", "GetAllHistos", "ReadFiFo", "WriteStatus", "Resize", "EnableControls", "DisableControls", "Error", "Exit"]
        # "100 x 60 x 60 x 1000 = 100 h"
        # "Init all FP controls and corresponding copy in UIThread Data cluster"
        # "EnQ list of commands"
        # "Array with Inp.Chan."
        # "Initialization: 1. Init HW -> get # of channels -> make array for Inp.Channels\n2. Init all FP controls and corresponding fields in UIThread Data cluster\n3. EnQ list of commands for further initialization"
        n139 = disable-structure shown="TARGET_TYPE==Windows, Default" {
          disable-tunnel: ["MHLib64" ("name or relative path") "MHLib" ("name or relative path")] -> w314
          frame condition #0 (active) {
          }
          frame condition #1 {
          }
        }
        n140 = xnode "Error Ring"() -> ("error out"=w318:errorcluster)
        n141 = call "GetDLLPath.vi"("DllName_32bit"="MHLib" ("name or relative path"), "DllName_64bit"=w314) -> ("file exists?"=w320:bool, "DLLPath"=w321:path)  [unwired: 8 in]
        n142 = global write "MH_DllPath_global.vi" "DllPath"(w321) -> ()
        n143 = property on="AllChannels" class="Clust (strict)"("Val(Sgnl)"=T1 {"Enable"=TRUE, "Offset"=0, "Level"=-100, "Edge"=0, "DeadTime"=1000, "UseDeadTime"=FALSE, "SetEnableAllChan"=TRUE, "SetEdgeAllChan"=TRUE, "SetLevelAllChan"=TRUE, "SetOffsetAllChan"=TRUE, "SetUseDTAllChan"=TRUE, "SetDeadTAllChan"=TRUE} ("AllChannels")) -> ()  [unwired: 2 in, 2 out]
        n144 = Select(t=errorcluster {"status"=FALSE, "code"=0, "source"=""} ("error IO"), s=w320, f=w318) -> (s? t:f=w335:errorcluster)
        n145 = global read "MH_LibVersion_global.vi" "Library Version"() -> (w316:string)
        n146 = Build Array (concatenate)(w355, w354) -> (w353:T13[])
        n147 = call "InitMH_UIThread.vi"("error in (no error)"=w335, "Mode"=w315, "refsource"=w317, "Library Version"=w316) -> ("error out"=w356:errorcluster, "Init Info"=w358:T10, "DevIdx"=w357:i32)  [unwired: 5 in]
        n148 = local write "SyncDivider"(w352) -> ()
        n149 = local write "SyncOffset"(w351) -> ()
        n150 = local write "SyncEdge"(w350) -> ()
        n151 = local write "SyncLevel"(w349) -> ()
        n152 = local write "Binning"(w348) -> ()
        n153 = Bundle By Name(cluster=w339, "DevIdx"=w357, "Init Info"=w358, "Status"="Initialized!") -> (w338:T9)
        n154 = Unbundle By Name(w338) -> ("Init Info.Bin Steps"=w337:i32, "Init Info.nchannels"=w311:i32)
        n155 = for {
          N: w311 -> [_]
          i -> [w366]
          n156 = Increment(x=w366) -> (x+1=w369:i32)
          n157 = Format Into String(format string="Ch.%d", w369) -> (resulting string=w367:string)  [unwired: 2 in, 1 out]
          n158 = property on="HistoGraph" class="WFGraph (strict)"("Active Plot"=w366, "Plot.Plot Name"=w367) -> ()  [unwired: 2 in, 2 out]
          n159 = property on="TTraceGraph" class="WFGraph (strict)"("Active Plot"=w366, "Plot.Plot Name"=w367) -> ()  [unwired: 2 in, 2 out]
        }
        n160 = Bundle By Name(cluster=T6 {"Histos"=[], "Cmd"=enum."_none_", "TimeTrace"=[], "Bin"=0, "Total bin"=0, "Status"="", "Resol"=0.0, "DeltaT"=0.0, "nChannels"=0} ("MH_GUIThread_QData"), "Cmd"=MH_VisThread_QCmds."nChannels", "nChannels"=w311) -> (w327:T6)
        n161 = call "MH_CalcBinningValues.vi"("Bin Steps"=w337) -> ("BinningValues"=w342:cluster{"String":string, "Value":i32}[])  [unwired: 10 in]
        n162 = call "MH_InitChannels.vi"("nchannels"=w311) -> ("SetInpChan"=w309:T11[], "Channels"=w310:T3[])  [unwired: 9 in]
        n163 = property on="Binning" class="Ring (strict)"("StringsAndValues[]"=w342) -> ()  [unwired: 2 in, 2 out]
        n164 = Bundle By Name(cluster=T8 {"Cmd"=enum."Proc", "nActual"=0, "Buffer"=[], "TickCount"=0, "Param"=0} ("MH_DataProcThread_QData"), "Param"=w311, "Cmd"=MH_DataProcThread_QCmds."SetNumChannels") -> (w331:T8)
        n165 = Enqueue Element(queue=w325, element=w327) -> ()  [unwired: 2 in, 3 out]
        n166 = Enqueue Element(queue=w332, element=w331) -> ()  [unwired: 2 in, 3 out]
        n167 = local write "Channels"(w310) -> ()
        n168 = Bundle By Name(cluster=w338, "Channels"=w310, "SetInpChan"=w309, "SyncDivider"=w352, "SyncOffset"=w351, "SyncEdge"=w350, "SyncLevel"=w349, "Binning"=w348, "HistoOffset"=w347, "AcqTime"=w346, "StopOvl."=w345, "OvlLevel"=w344, "StartMeas"=w343, "Run cont."=w341, "BitShift"=w324, "HistoAcqTime"=w323, "UseDeadTime"=w313, "SyncDeadTime"=w312) -> (w334:T9)
        n169 = local write "AcqTime"(w346) -> ()
        n170 = local write "StopOvl."(w345) -> ()
        n171 = local write "OvlLevel"(w344) -> ()
        n172 = local write "Start"(w343) -> ()
        n173 = local write "Run continuously"(w341) -> ()
        n174 = local write "BitShift"(w324) -> ()
        n175 = local write "HistoAcqTime"(w323) -> ()
        n176 = local write "HistoOffset"(w347) -> ()
        n177 = local write "UseDeadTime"(w313) -> ()
        n178 = local write "SyncDeadTime"(w312) -> ()
        n179 = property on="Settings" class="Bool (strict)"("Val(Sgnl)"=TRUE ("Value (Signaling)")) -> ()  [unwired: 2 in, 2 out]
        n180 = property on="Scale" class="Bool (strict)"("Val(Sgnl)"=FALSE ("Value (Signaling)")) -> ()  [unwired: 2 in, 2 out]
      }
      frame "SetInpChan" {
        n181 = Unbundle By Name(w377) -> ("DevIdx"=w375:i32, "Init Info.features"=w374:i32, "SetInpChan"=w373:T11[], "Channels"=w372:T3[])
        n182 = for {
          tunnel: w372 -> [w382]
          tunnel: w373 -> [w386] mode=indexing
          shift-right: [w384] -> w371
          shift-left: errorcluster {"status"=FALSE, "code"=0, "source"=""} ("error out") -> [w383]
          tunnel: w375 -> [w380]
          tunnel: w374 -> [w378]
          n183 = Unbundle By Name(w386) -> ("Cmds"=w385:T12[], "Channel"=w379:i32)
          n184 = Index Array(array=w382, index=w379) -> (element=w381:T3)
          n185 = for {
            tunnel: w385 -> [w393] mode=indexing
            tunnel: w379 -> [w392]
            shift-right: [w391] -> w384
            shift-left: w383 -> [w390]
            tunnel: w381 -> [w389]
            tunnel: w380 -> [w388]
            tunnel: w378 -> [w387]
            n186 = case shown="\"SetInpChanDeadTime\"" w393 {
              tunnel: w392 -> [_ w399 w406 w411 w427]
              tunnel: [w394 w398 w405 w415 w432] -> w391
              tunnel: w390 -> [w394 w397 w404 w414 w431]
              tunnel: w389 -> [_ w396 w403 w413 w430]
              tunnel: w388 -> [_ w395 w402 w412 w429]
              tunnel: w387 -> [_ _ _ w408 _]
              frame Default {
              }
              frame "SetInpChanEnable" {
                n187 = Unbundle By Name(w396) -> ("Enable"=w400:bool)
                n188 = call "MH_SetInputChannelEnable.vi"("error in (no error)"=w397, "enable"=w400, "channel"=w399, "devidx"=w395) -> ("error out"=w398:errorcluster)  [unwired: 6 in, 1 out]
              }
              frame "SetInpChanOffset" {
                n189 = Unbundle By Name(w403) -> ("Offset"=w401:i32)
                n190 = call "MH_SetInputChannelOffset.vi"("error in (no error)"=w404, "Offset"=w401, "channel"=w406, "devidx"=w402) -> ("error out"=w405:errorcluster)  [unwired: 6 in, 1 out]
              }
              frame "SetInpChanDeadTime" {
                w409 = 32  # FEATURE_PROG_TD
                n191 = And(x=w408, y=w409) -> (x .and. y?=w410:i32)
                n192 = Not Equal To 0?(x=w410) -> (x != 0?=w407:bool)
                n193 = case shown="False" w407 {
                  tunnel: [w416 w425] -> w415
                  tunnel: w414 -> [w416 w424]
                  tunnel: w413 -> [_ w423]
                  tunnel: w412 -> [_ w422]
                  tunnel: w411 -> [_ w420]
                  frame False {
                  }
                  frame True {
                    n194 = Unbundle By Name(w423) -> ("UseDeadTime"=w419:bool, "DeadTime"=w421:i32)
                    n195 = Boolean To (0,1)(Boolean=w419) -> (0, 1=w418:i16)
                    n196 = To Long Integer(number=w418) -> (32bit integer=w417:i32)
                    n197 = call "MH_SetInputDeadTime.vi"("channel"=w420, "error in (no error)"=w424, "deadtime"=w421, "on"=w417, "devidx"=w422) -> ("error out"=w425:errorcluster)  [unwired: 5 in, 1 out]
                  }
                }
              }
              frame "SetInpChanTrg" {
                n198 = Unbundle By Name(w430) -> ("Level"=w426:i32, "Edge"=w428:i32)
                n199 = call "MH_SetInputEdgeTrg.vi"("channel"=w427, "error in (no error)"=w431, "edge"=w428, "level"=w426, "devidx"=w429) -> ("error out"=w432:errorcluster)  [unwired: 5 in, 1 out]
              }
            }
          }
        }
      }
      frame "SetSyncDivider" {
        n200 = Unbundle By Name(w440) -> ("DevIdx"=w439:i32, "SyncDivider"=w435:i32)
        n201 = Power Of 2(x=w435) -> (2^x=w434:dbl)
        n202 = To Long Integer(number=w434) -> (32bit integer=w433:i32)
        n203 = call "MH_SetSyncDiv.vi"("SyncDivider"=w433, "devidx"=w439) -> ("error out"=w437:errorcluster)  [unwired: 8 in, 1 out]
        n204 = flat-sequence {
          tunnel: w437 -> [w441]
          tunnel: [w441] -> w436
          frame #0 {
            n205 = Wait (ms)(milliseconds to wait=u32 100) -> ()  [unwired: 1 out]
          }
        }
      }
      frame "SetSyncTrg" {
        n206 = Unbundle By Name(w448) -> ("DevIdx"=w445:i32, "SyncLevel"=w443:i32, "SyncEdge"=w444:i32)
        n207 = call "MH_SetSyncEdgeTrg.vi"("edge"=w444, "level"=w443, "devidx"=w445) -> ("error out"=w446:errorcluster)  [unwired: 7 in, 1 out]
      }
      frame "SetSyncDeadTime" {
        w451 = 32  # FEATURE_PROG_TD
        n208 = Unbundle By Name(w460) -> ("DevIdx"=w457:i32, "UseDeadTime"=w454:bool, "SyncDeadTime"=w456:i32, "Init Info.features"=w450:i32)
        n209 = And(x=w450, y=w451) -> (x .and. y?=w452:i32)
        n210 = Boolean To (0,1)(Boolean=w454) -> (0, 1=w455:i16)
        n211 = Not Equal To 0?(x=w452) -> (x != 0?=w449:bool)
        n212 = To Long Integer(number=w455) -> (32bit integer=w453:i32)
        n213 = case shown="True" w449 {
          tunnel: [_ w464] -> w458
          tunnel: w457 -> [_ w463]
          tunnel: w456 -> [_ w462]
          tunnel: w453 -> [_ w461]
          frame False {
          }
          frame True {
            n214 = call "MH_SetSyncDeadTime.vi"("deadtime"=w462, "on"=w461, "devidx"=w463) -> ("error out"=w464:errorcluster)  [unwired: 7 in, 1 out]
          }
        }
      }
      frame "SetSyncOffset" {
        n215 = Unbundle By Name(w469) -> ("DevIdx"=w467:i32, "SyncOffset"=w466:i32)
        n216 = call "MH_SetSyncChannelOffset.vi"("Offset"=w466, "devidx"=w467) -> ("error out"=w468:errorcluster)  [unwired: 8 in, 1 out]
      }
      frame "SetBinning" {
        # "When binning is changed the new resolution is querried"
        n217 = Unbundle By Name(w476) -> ("DevIdx"=w474:i32, "Binning"=w473:i32)
        n218 = call "MH_SetBinning.vi"("Binning"=w473, "devidx"=w474) -> ("error out"=w475:errorcluster)  [unwired: 8 in, 1 out]
        n219 = Build Array (concatenate)(MH_UIThread_Cmds."GetResolution", w471) -> (w472:T13[])
      }
      frame "SetHistoOffset" {
        n220 = Unbundle By Name(w481) -> ("DevIdx"=w478:i32, "HistoOffset"=w477:i32)
        n221 = call "MH_SetOffset.vi"("Offset"=w477, "devidx"=w478) -> ("error out"=w479:errorcluster)  [unwired: 8 in, 1 out]
      }
      frame "SetStopOvl" {
        n222 = Unbundle By Name(w488) -> ("DevIdx"=w485:i32, "StopOvl."=w484:bool, "OvlLevel"=w483:u32)
        n223 = To Unsigned Long Integer(number=w483) -> (unsigned 32bit integer=w482:u32)
        n224 = call "MH_SetStopOverflow.vi"("stopcount"=w482, "StopOnOverflow"=w484, "devidx"=w485) -> ("error out"=w486:errorcluster)  [unwired: 7 in, 1 out]
      }
      frame "SetBitShift" {
        n225 = Unbundle By Name(w492) -> ("BitShift"=w490:i32, "SyncRate"=w491:i32)
        n226 = Negate(x=w490) -> (-x=w500:i32)
        n227 = Bundle By Name(cluster=T8 {"Cmd"=enum."Proc", "nActual"=0, "Buffer"=[], "TickCount"=0, "Param"=0} ("MH_DataProcThread_QData"), "Param"=w500, "Cmd"=MH_DataProcThread_QCmds."SetShift") -> (w506:T8)
        n228 = To Double Precision Float(number=w490) -> (double precision float=w505:dbl)
        n229 = To Double Precision Float(number=w491) -> (double precision float=w504:dbl)
        n230 = Power Of 2(x=w505) -> (2^x=w503:dbl)
        n231 = Enqueue Element(queue=w493, element=w506) -> ()  [unwired: 2 in, 3 out]
        n232 = Multiply(x=w503, y=1000.0) -> (x*y=w502:dbl)
        n233 = Divide(x=w502, y=w504) -> (x/y=w489:dbl)
        "DeltaT" <- w489
        n234 = Bundle By Name(cluster=T6 {"Histos"=[], "Cmd"=enum."_none_", "TimeTrace"=[], "Bin"=0, "Total bin"=0, "Status"="", "Resol"=0.0, "DeltaT"=0.0, "nChannels"=0} ("MH_GUIThread_QData"), "DeltaT"=w489, "Cmd"=MH_VisThread_QCmds."DeltaT") -> (w501:T6)
        n235 = Enqueue Element(queue=w494, element=w501) -> ()  [unwired: 2 in, 3 out]
      }
      frame "SetHistoAcqTime" {
        n236 = Unbundle By Name(w509) -> ("SyncRate"=w515:i32, "HistoAcqTime"=w508:dbl)
        n237 = To Double Precision Float(number=w515) -> (double precision float=w518:dbl)
        n238 = Multiply(x=w518, y=w508) -> (x*y=w517:dbl)
        n239 = Round To Nearest(number=w517) -> (nearest integer value=w516:dbl)
        n240 = To Long Integer(number=w516) -> (32bit integer=w514:i32)
        n241 = Bundle By Name(cluster=T8 {"Cmd"=enum."Proc", "nActual"=0, "Buffer"=[], "TickCount"=0, "Param"=0} ("MH_DataProcThread_QData"), "Param"=w514, "Cmd"=MH_DataProcThread_QCmds."SetHistAcqTime") -> (w513:T8)
        n242 = Enqueue Element(queue=w510, element=w513) -> ()  [unwired: 2 in, 3 out]
      }
      frame "GetAllRates" {
        # "An alternative to GetRates"
        n243 = Unbundle By Name(w521) -> ("DevIdx"=w529:i32, "Init Info.nchannels"=w536:i32, "StartMeas"=w530:bool, "SyncRateStart"=w524:i32)
        n244 = call "MH_AllocateCntRateBuffer.vi"("NumChan"=w536) -> ("Buffer"=w535:i32[])  [unwired: 10 in]
        n245 = call "MH_GetAllCountRates.vi"("cntrates_buf"=w535, "devidx"=w529) -> ("error out"=w528:errorcluster, "cntrates"=→"CountRates":i32[], "syncrate"=w526:i32)  [unwired: 6 in, 1 out]
        n246 = case shown="True" w530 {
          tunnel: w529 -> [_ w551]
          tunnel: w528 -> [w540 w550]
          tunnel: [w540 w549] -> w527
          tunnel: w526 -> [w539 _]
          tunnel: [w539 w546] -> w525
          tunnel: w524 -> [_ w541]
          tunnel: w523 -> [w538 w545]
          tunnel: [w538 w544] -> w522
          tunnel: w521 -> [w537 w543]
          tunnel: [w537 w542] -> w520
          frame False {
          }
          frame True {
            n247 = call "MH_GetSyncPeriod.vi"("error in (no error)"=w550, "devidx"=w551) -> ("error out"=w549:errorcluster, "period"=w548:dbl)  [unwired: 7 in, 1 out]
            n248 = Reciprocal(x=w548) -> (1/x=w547:dbl)
            n249 = To Long Integer(number=w547) -> (32bit integer=w546:i32)
            n250 = case shown="-1" w541 {
              selector: w541 -> [w552 _ _]
              tunnel: w546 -> [w555 w576 _]
              tunnel: w545 -> [w553 w578 w582]
              tunnel: [w554 w578 w582] -> w544
              tunnel: w543 -> [w559 w577 w581]
              tunnel: [w559 w575 w580] -> w542
              frame Default {
                n251 = Subtract(x=w555, y=w552) -> (x-y=w558:i32)
                n252 = Absolute Value(x=w558) -> (abs(x)=w556:i32)
                n253 = Not Equal To 0?(x=w556) -> (x != 0?=w557:bool)
                n254 = case shown="True" w557 {
                  tunnel: w556 -> [_ w568]
                  tunnel: [w560 w563] -> w554
                  tunnel: w553 -> [w560 w562]
                  tunnel: w552 -> [_ w561]
                  frame False {
                  }
                  frame True {
                    n255 = To Double Precision Float(number=w568) -> (double precision float=w567:dbl)
                    n256 = To Double Precision Float(number=w561) -> (double precision float=w569:dbl)
                    n257 = Divide(x=w567, y=w569) -> (x/y=w566:dbl)
                    n258 = Greater Or Equal?(x=w566, y=0.01) -> (x >= y?=w564:bool)
                    n259 = case shown="False" w564 {
                      tunnel: [w570 w573] -> w563
                      tunnel: w562 -> [w570 w571]
                      frame False {
                      }
                      frame True {
                        w572 = T13[] [enum."StopMeas"] items=["Idle", "Init", "SetInpChan", "SetSyncDivider", "SetSyncTrg", "SetSyncOffset", "SetSyncDeadTime", "SetBinning", "SetHistoOffset", "SetHistoLen", "SetStopOvl", "SetBitShift", "SetHistoAcqTime", "GetRates", "GetAllRates", "StartMeas", "StopMeas", "AbortMeas", "GetResolution", "GetHistos", "GetAllHistos", "ReadFiFo", "WriteStatus", "Resize", "EnableControls", "DisableControls", "Error", "Exit"]
                        n260 = One Button Dialog(message="Warning: Sync Rate has changed!\nTime Trace resolution has been changed accordingly.\nMeasurement is aborted.\n") -> ()  [unwired: 1 in, 1 out]
                        n261 = Build Array (concatenate)(w571, w572) -> (w573:T13[])
                      }
                    }
                  }
                }
              }
              frame -1 {
                n262 = Bundle By Name(cluster=w577, "SyncRateStart"=w576) -> (w575:T9)
              }
              frame -2 {
                n263 = Bundle By Name(cluster=w581, "SyncRateStart"=-1) -> (w580:T9)
              }
            }
          }
        }
        n264 = Bundle By Name(cluster=w520, "SyncRate"=w525) -> (w531:T9)
        n265 = Format Into String(format string="Sync Rate: %d cps\n", w525) -> (resulting string=→"SyncRate":string)  [unwired: 2 in, 1 out]
      }
      frame "GetRates" {
        # "An alternative to GetAllRates"
        n266 = Unbundle By Name(w587) -> ("Init Info.nchannels"=w592:i32, "Channels"=w588:T3[], "DevIdx"=w589:i32)
        n267 = call "MH_GetSyncRate.vi"("devidx"=w589) -> ("error out"=w591:errorcluster, "syncrate"=w585:i32)  [unwired: 8 in, 1 out]
        n268 = Format Into String(format string="Sync Rate: %d cps\n", w585) -> (resulting string=w584:string)  [unwired: 2 in, 1 out]
        n269 = local write "SyncRate"(w584) -> ()
        n270 = for {
          N: w592 -> [_]
          tunnel: w589 -> [w600]
          tunnel: [w597] -> w583 mode=indexing
          shift-right: [w599] -> w593
          shift-left: w591 -> [w601]
          tunnel: w588 -> [w596] mode=indexing
          i -> [w598]
          n271 = Unbundle By Name(w596) -> ("Enable"=w595:bool)
          n272 = case shown="True" w595 {
            tunnel: w601 -> [w602 w607]
            tunnel: w600 -> [_ w606]
            tunnel: [w602 w605] -> w599
            tunnel: w598 -> [_ w604]
            tunnel: [_ w603] -> w597
            frame False {
            }
            frame True {
              n273 = call "MH_GetCountRate.vi"("error in (no error)"=w607, "Channel"=w604, "devidx"=w606) -> ("error out"=w605:errorcluster, "rate"=w603:i32)  [unwired: 6 in, 1 out]
            }
          }
        }
        n274 = local write "CountRates"(w583) -> ()
        n275 = Bundle By Name(cluster=w587, "SyncRate"=w585) -> (w586:T9)
      }
      frame "StartMeas" {
        n276 = Bundle By Name(cluster=T8 {"Cmd"=enum."Proc", "nActual"=0, "Buffer"=[], "TickCount"=0, "Param"=0} ("MH_DataProcThread_QData"), "Cmd"=MH_DataProcThread_QCmds."Init") -> (w612:T8)
        n277 = Unbundle By Name(w610) -> ("DevIdx"=w619:i32, "AcqTime"=w615:i32)
        n278 = Enqueue Element(queue=w614, element=w612) -> ()  [unwired: 2 in, 3 out]
        n279 = Bundle By Name(cluster=w610, "SyncRateStart"=-2) -> (w609:T9)
        n280 = call "MH_StartMeas.vi"("tacq"=w615, "devidx"=w619) -> ("error out"=w620:errorcluster)  [unwired: 8 in, 1 out]
        n281 = Build Array (concatenate)(w618, MH_UIThread_Cmds."ReadFiFo") -> (w617:T13[])
      }
      frame "StopMeas" {
        n282 = Unbundle By Name(w626) -> ("Run cont."=w621:bool, "DevIdx"=w627:i32)
        n283 = call "MH_StopMeas.vi"("devidx"=w627) -> ("error out"=w628:errorcluster)  [unwired: 9 in, 1 out]
        n284 = case shown="False" w621 {
          tunnel: w626 -> [w632 w634]
          tunnel: [w631 w634] -> w625
          tunnel: [w629 w633] -> w624
          frame False {
            w629 = T13[] [enum."ReadFiFo"] items=["Idle", "Init", "SetInpChan", "SetSyncDivider", "SetSyncTrg", "SetSyncOffset", "SetSyncDeadTime", "SetBinning", "SetHistoOffset", "SetHistoLen", "SetStopOvl", "SetBitShift", "SetHistoAcqTime", "GetRates", "GetAllRates", "StartMeas", "StopMeas", "AbortMeas", "GetResolution", "GetHistos", "GetAllHistos", "ReadFiFo", "WriteStatus", "Resize", "EnableControls", "DisableControls", "Error", "Exit"]
            w630 = FALSE ("StartMeas")
            n285 = Bundle By Name(cluster=w632, "StartMeas"=w630) -> (w631:T9)
            n286 = local write "Start"(w630) -> ()
          }
          frame True {
            w633 = T13[] [enum."ReadFiFo", enum."StartMeas"] items=["Idle", "Init", "SetInpChan", "SetSyncDivider", "SetSyncTrg", "SetSyncOffset", "SetSyncDeadTime", "SetBinning", "SetHistoOffset", "SetHistoLen", "SetStopOvl", "SetBitShift", "SetHistoAcqTime", "GetRates", "GetAllRates", "StartMeas", "StopMeas", "AbortMeas", "GetResolution", "GetHistos", "GetAllHistos", "ReadFiFo", "WriteStatus", "Resize", "EnableControls", "DisableControls", "Error", "Exit"]
          }
        }
        n287 = Build Array (concatenate)(w623, w624) -> (w622:T13[])
      }
      frame "AbortMeas" {
        w636 = FALSE ("StartMeas")
        n288 = Unbundle By Name(w638) -> ("DevIdx"=w639:i32)
        n289 = call "MH_StopMeas.vi"("devidx"=w639) -> ("error out"=w640:errorcluster)  [unwired: 9 in, 1 out]
        n290 = Bundle By Name(cluster=w638, "StartMeas"=w636) -> (w637:T9)
        n291 = local write "Start"(w636) -> ()
      }
      frame "GetResolution" {
        # "Resolution in ns"
        # "Gets resolution in ps"
        # "Resolution is saved in UIThread Data cluster in ns"
        n292 = Unbundle By Name(w649) -> ("DevIdx"=w651:i32)
        n293 = call "MH_GetResolution.vi"("devidx"=w651) -> ("error out"=w650:errorcluster, "resolution"=w647:dbl)  [unwired: 8 in, 1 out]
        n294 = Divide(x=w647, y=1000.0) -> (x/y=w643:dbl)
        n295 = Bundle By Name(cluster=w649, "Resolution"=w643) -> (w648:T9)
        n296 = Bundle By Name(cluster=T6 {"Histos"=[], "Cmd"=enum."_none_", "TimeTrace"=[], "Bin"=0, "Total bin"=0, "Status"="", "Resol"=0.0, "DeltaT"=0.0, "nChannels"=0} ("MH_GUIThread_QData"), "Resol"=w643, "Cmd"=MH_VisThread_QCmds."Resol") -> (w641:T6)
        n297 = Enqueue Element(queue=w645, element=w641) -> ()  [unwired: 2 in, 3 out]
      }
      frame "ReadFiFo" {
        w661 = 2  # FLAG_FIFOFULL
        # "Reads photon records from HW and transferes them to DataProcThread via Queue."
        n298 = Unbundle By Name(w663) -> ("DevIdx"=w657:i32)
        n299 = call "MH_GetFlags.vi"("devidx"=w657) -> ("error out"=w659:errorcluster, "flags"=w660:i32)  [unwired: 8 in, 1 out]
        n300 = And(x=w660, y=w661) -> (x .and. y?=w662:i32)
        n301 = Not Equal To 0?(x=w662) -> (x != 0?=w656:bool)
        "OverRun" <- w656
        n302 = case shown="False" w656 {
          tunnel: w659 -> [w673 w676]
          tunnel: [w672 w676] -> w658
          tunnel: w657 -> [w665 _]
          tunnel: w655 -> [w671 _]
          tunnel: w654 -> [w670 _]
          tunnel: [w670 w674] -> w653
          frame False {
            n303 = call "MH_ReadFiFo.vi"("error in (no error)"=w673, "devidx"=w665) -> ("error out"=w672:errorcluster, "nactual"=w664:i32, "buffer"=w668:u32[])  [unwired: 6 in, 1 out]
            n304 = Bundle By Name(cluster=T8 {"Cmd"=enum."Proc", "nActual"=0, "Buffer"=[], "TickCount"=0, "Param"=0} ("MH_DataProcThread_QData"), "Buffer"=w668, "nActual"=w664, "Cmd"=MH_DataProcThread_QCmds."Proc") -> (w666:T8)
            n305 = Enqueue Element(queue=w671, element=w666) -> ()  [unwired: 2 in, 3 out]
          }
          frame True {
            n306 = Build Array(MH_UIThread_Cmds."AbortMeas") -> (w674:T13[])
          }
        }
      }
      frame "WriteStatus" {
        n307 = Unbundle By Name(w678) -> ("Status"=→"Status":string)
      }
      frame "Resize" {
        n308 = property on="Pane 3" class="Pane"() -> ("Width"=w685:u32)  [unwired: 2 in, 2 out]
        n309 = Subtract(x=w685, y=i16 100 ("b")) -> (x-y=w691:u32)
        n310 = Unbundle By Name(w680) -> ("Init Info.nchannels"=w688:i32)
        n311 = Quotient & Remainder(x=w691, y=i16 99 ("m")) -> (floor(x/y)=w690:u32)  [unwired: 1 out]
        n312 = In Range and Coerce(upper limit=w688, x=w690, lower limit=4) -> (coerced(x)=w689:u32)  [unwired: 1 out]
        n313 = Equal?(x=w688, y=w689) -> (x = y?=w687:bool)
        n314 = Not(x=w687) -> (.not. x?=w686:bool)
        n315 = property on="Channels" class="Arr (strict)"("HorizScroll"=w686, "Number of Columns"=w689, "Index Values"=u32[] [0]) -> ()  [unwired: 2 in, 2 out]
      }
      frame "EnableControls" {
        n316 = property class="VI"() -> ("Panel"=w696:refnum<vi>)  [unwired: 2 in, 2 out]
        n317 = property class="Pnl"(reference=w696) -> ("Controls[]"=w695:refnum<vi>[])  [unwired: 1 in, 2 out]
        n318 = property class="Pnl"(reference=w696) -> ("Decos[]"=w697:refnum<vi>[])  [unwired: 1 in, 2 out]
        n319 = for {
          tunnel: w697 -> [w701] mode=indexing
          tunnel: TRUE -> [w700]
          n320 = property class="Decor"(reference=w701, "Visible"=w700) -> ()  [unwired: 1 in, 2 out]
        }
        n321 = for {
          tunnel: w695 -> [w704] mode=indexing
          tunnel: T14."Enabled" ("Disabled") -> [w703]
          tunnel: [w702] -> _
          n322 = property class="Ctl"(reference=w704, "DisabledEnum"=w703) -> (error out=w702:errorcluster)  [unwired: 1 in, 1 out]
        }
      }
      frame "DisableControls" {
        n323 = property class="VI"() -> ("Panel"=w708:refnum<vi>)  [unwired: 2 in, 2 out]
        n324 = property class="Pnl"(reference=w708) -> ("Controls[]"=w707:refnum<vi>[])  [unwired: 1 in, 2 out]
        n325 = property class="Pnl"(reference=w708) -> ("Decos[]"=w709:refnum<vi>[])  [unwired: 1 in, 2 out]
        n326 = for {
          tunnel: w709 -> [w713] mode=indexing
          tunnel: FALSE -> [w712]
          n327 = property class="Decor"(reference=w713, "Visible"=w712) -> ()  [unwired: 1 in, 2 out]
        }
        n328 = for {
          tunnel: w707 -> [w716] mode=indexing
          tunnel: T14."Disabled and Grayed Out" ("Disabled") -> [w715]
          tunnel: [w714] -> _
          n329 = property class="Ctl"(reference=w716, "DisabledEnum"=w715) -> (error out=w714:errorcluster)  [unwired: 1 in, 1 out]
        }
      }
      frame "Error" {
        w717 = T13[] [enum."Exit"] items=["Idle", "Init", "SetInpChan", "SetSyncDivider", "SetSyncTrg", "SetSyncOffset", "SetSyncDeadTime", "SetBinning", "SetHistoOffset", "SetHistoLen", "SetStopOvl", "SetBitShift", "SetHistoAcqTime", "GetRates", "GetAllRates", "StartMeas", "StopMeas", "AbortMeas", "GetResolution", "GetHistos", "GetAllHistos", "ReadFiFo", "WriteStatus", "Resize", "EnableControls", "DisableControls", "Error", "Exit"]
        w720 = T18 1 items=["no dialog", "OK message", "continue or stop message", "OK message + warnings", "continue/stop + warnings"] ("type of dialog (OK msg:1)")
        # "Error case: If an error occures the user is informed and the programm terminates. Add your own code to handle error events (e.g. exception lists, etc.)"
        n330 = call <vilib>:"Simple Error Handler.vi"("type of dialog (OK msg:1)"=w720, "error in (no error)"=w719) -> ()  [unwired: 3 in, 5 out]
      }
      frame "Exit" {
        n331 = Release Queue(queue=w722) -> ()  [unwired: 2 in, 3 out]
        n332 = Release Queue(queue=w721) -> ()  [unwired: 2 in, 3 out]
        n333 = Unbundle By Name(w726) -> ("DevIdx"=w725:i32)
        n334 = call "MH_CloseDevice.vi"("devidx"=w725) -> ("error out"=w724:errorcluster)  [unwired: 9 in, 1 out]
      }
    }
    n335 = call "MH_EnQError.vi"("error in (no error)"=w24, "Cmds_in"=w22) -> ("error out"=w23:errorcluster, "Cmds_out"=w21:T13[])  [unwired: 8 in]
  }
  n336 = call "MH_DataProcThread.vi"("MH_VisThread_QRef"=w7, "MH_DataProcThread_QRef"=w1) -> ()  [unwired: 10 in]
  n337 = while {
    tunnel: w7 -> [w735]
    shift-right: [w731] -> _
    shift-left: T5 {"Resol"=0.0, "DeltaT"=0.0, "NumChannels"=0} -> [w732]
    tunnel: w1 -> [w730]
    stop <- w728 stop-if-true
    # "VisualizationThread"
    n338 = Dequeue Element(queue=w735, timeout in ms (-1)=100) -> (element=w733:T6, error out=w728:errorcluster)  [unwired: 1 in, 2 out]
    n339 = Unbundle By Name(w733) -> ("Cmd"=w734:T7)
    n340 = case shown="\"TTrace\"" w734 {
      tunnel: w733 -> [_ w748 w750 w762 w770 w774 w778]
      tunnel: w732 -> [w738 w746 w752 w754 w769 w773 w777]
      tunnel: [w738 w746 w751 w754 w769 w772 w776] -> w731
      tunnel: w730 -> [w737 _ _ _ w766 _ _]
      tunnel: w728 -> [w736 _ _ _ _ _ _]
      frame "_none_", Default {
        n341 = case shown="No Error" w736 {
          tunnel: w737 -> [w742 _]
          frame No Error {
            n342 = Get Queue Status(queue=w742) -> (# elements in queue=w740:i32)  [unwired: 2 in, 7 out]
            n343 = Format Into String(format string="Elements in Q: %d", w740) -> (resulting string=w739:string)  [unwired: 2 in, 1 out]
            n344 = local write "Status"(w739) -> ()
          }
          frame Error {
          }
        }
      }
      frame "Histo" {
        n345 = Unbundle By Name(w748) -> ("Histos"=w743:u32[][])
        n346 = Unbundle By Name(w746) -> ("Resol"=w745:dbl)
        n347 = Bundle(0.0, "Resol"=w745, "Histos"=w743) -> (→"HistoGraph":cluster{dbl, "Resol":dbl, "Histos":u32[][]})  [unwired: 1 in]
      }
      frame "nChannels" {
        n348 = Unbundle By Name(w750) -> ("nChannels"=w749:i32)
        n349 = Bundle By Name(cluster=w752, "NumChannels"=w749) -> (w751:T5)
      }
      frame "TTrace" {
        n350 = Unbundle By Name(w762) -> ("Total bin"=w761:u64, "Bin"=w760:i32, "TimeTrace"=w759:u32[][])
        n351 = Unbundle By Name(w754) -> ("DeltaT"=w753:dbl)
        n352 = call "MH_TTraceToGraph.vi"("DeltaT"=w753, "TimeTrace"=w759, "Bin"=w760, "Total bin"=w761) -> ("TimeTrace_out"=w756:u32[][], "dt"=w757:dbl, "T0"=w758:dbl)  [unwired: 5 in]
        n353 = Bundle("T0"=w758, "dt"=w757, "TimeTrace_out"=w756) -> (→"TTraceGraph":T19)  [unwired: 1 in]
      }
      frame "Status" {
        n354 = Unbundle By Name(w770) -> ("Status"=w767:string)
        n355 = Get Queue Status(queue=w766) -> (# elements in queue=w765:i32)  [unwired: 2 in, 7 out]
        n356 = Format Into String(format string="\t\tElements in Q: %d", w765) -> (resulting string=w763:string)  [unwired: 2 in, 1 out]
        n357 = Concatenate Strings(w767, w763) -> (w768:string)
        n358 = local write "Status"(w768) -> ()
      }
      frame "DeltaT" {
        n359 = Unbundle By Name(w774) -> ("DeltaT"=w771:dbl)
        n360 = Bundle By Name(cluster=w773, "DeltaT"=w771) -> (w772:T5)
      }
      frame "Resol" {
        n361 = Unbundle By Name(w778) -> ("Resol"=w775:dbl)
        n362 = Bundle By Name(cluster=w777, "Resol"=w775) -> (w776:T5)
      }
    }
  }
